vi "1-8.vi"() -> ()   [LabVIEW 2022 SP3]
panel:
  in  "仪表":dbl(knob) scale=0.0..10.0
  in  "旋钮":dbl(knob) scale=0.0..2.0
  out "数值 7":dbl
  out "数值 6":dbl
  out "数值 5":dbl
  in  "数值 4":dbl
  in  "数值 3":dbl
  in  "数值 2":i8 format="%x"
  in  "数值":dbl
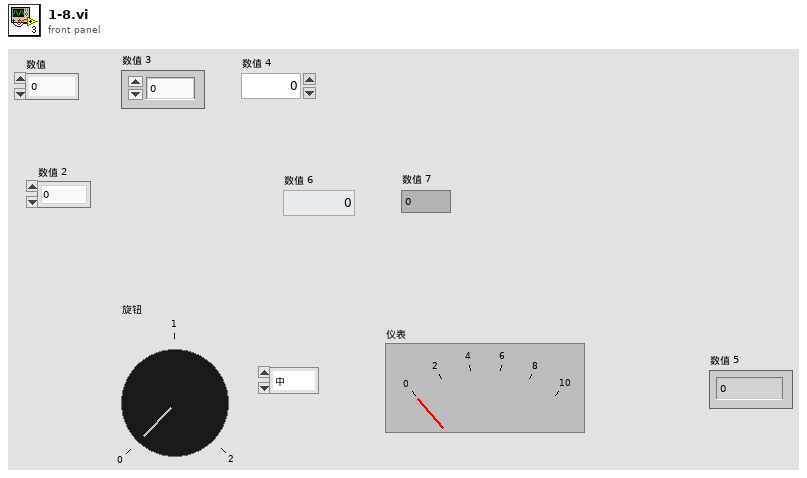
[diagram p1: front panel]
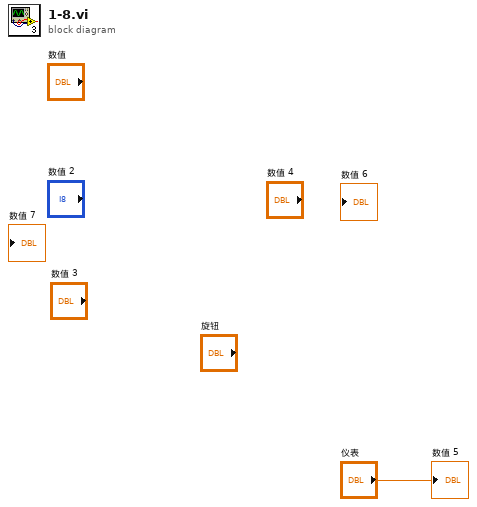
[diagram p0: block diagram]
diagram:
  "数值 5" <- "仪表"
